vi "SetSampleRate.vi"(8 "error in (no error)":errorcluster, 10 "SampleRate":dbl, 11 "ArbitraryFunction in":refnum<class "ArbitraryFunction.lvclass">) -> (0 "error out":errorcluster, 3 "ArbitraryFunction out":refnum<class "ArbitraryFunction.lvclass">)   [LabVIEW 2018, in "Functions.lvlib" / "ArbitraryFunction.lvclass"]
doc: "IVI Fgen standard does not provide for sample rate contrl, but many of the sub classes need ti so this provides an overridable method to input sample rate."
uses:
  ArbitraryFunction.lvclass
  ArbitraryFunction.lvclass/ArbitraryFunction.ctl
  Accessors/Write SampleRate.vi
panel:
  # "IVI Fgen standard does not provide for sample rate contrl, but many of the sub classes need ti so this provides an overridable method to input sample rate."
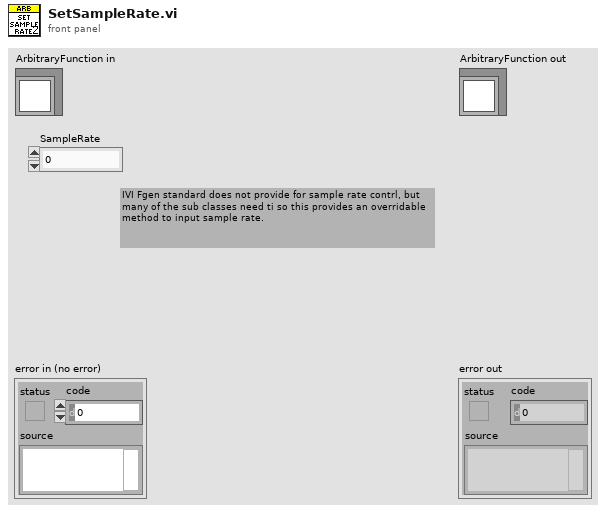
[diagram p1: front panel]
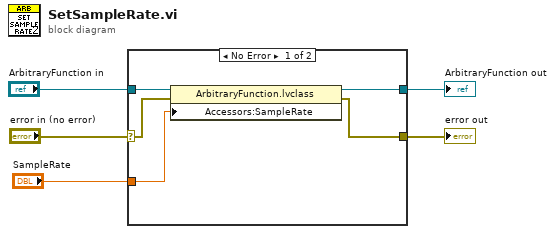
[diagram p0: block diagram]
diagram:
  n1 = case shown="No Error" "error in (no error)" {
    selector: "error in (no error)" -> [w9 w12]
    tunnel: [w6 w12] -> w4
    tunnel: "ArbitraryFunction in" -> [w10 w11]
    tunnel: [w7 w11] -> w2
    tunnel: "SampleRate" -> [w8 _]
    frame No Error {
      n2 = property class="ArbitraryFunction.lvclass"(reference=w10, error in=w9, "Accessors:SampleRate"=w8) -> (reference out=w7:refnum<class "ArbitraryFunction.lvclass">, error out=w6:errorcluster)
    }
    frame Error {
    }
  }
  "error out" <- w4
  "ArbitraryFunction out" <- w2
